vi "Helper - Best Tack Pt.vi"(10 "Point on Line":dbl[][](array[numeric]), 11 "Vector In":T1) -> (3 "Array":dbl[](array[numeric]))   [LabVIEW 2011]
uses:
  2 Typedefs/Velocity.ctl
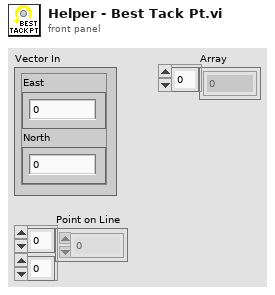
[diagram p1: front panel]
types:
  T1 = typedef "Velocity.ctl" = cluster{"East":dbl, "North":dbl}
  T2 = typedef "heading.ctl" = dbl
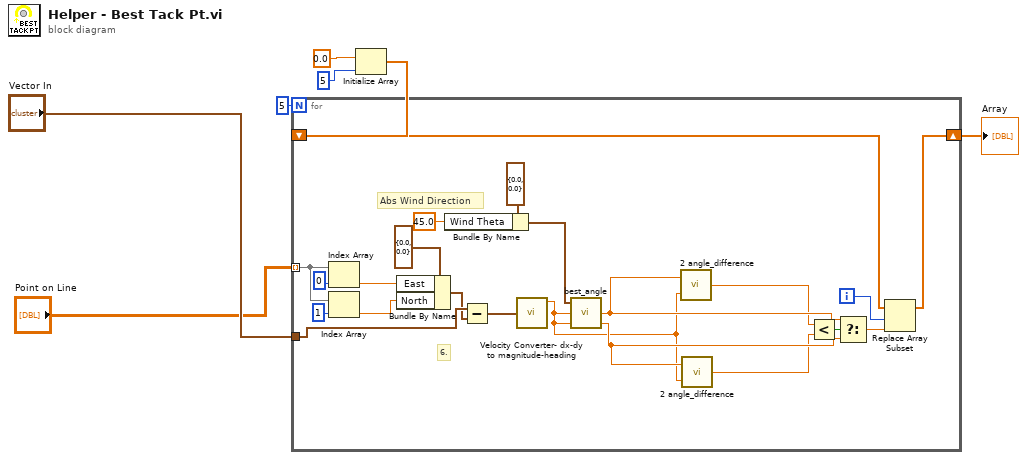
[diagram p0: block diagram]
diagram:
  n1 = Initialize Array(0.0, 5) -> (w4:dbl[])
  n2 = for {
    N: 5 -> [_]
    tunnel: "Vector In" -> [w23]
    tunnel: "Point on Line" -> [w29] mode=indexing
    shift-right: [w14] -> w5
    shift-left: w4 -> [w16]
    i -> [w15]
    # "6."
    # "Abs Wind Direction"
    n3 = Index Array(array=w29, index=0) -> (element=w25:dbl)
    n4 = Index Array(array=w29, index=1) -> (element=w24:dbl)
    n5 = Bundle By Name(cluster=T1 {"East"=0.0, "North"=0.0} ("Vector In"), "East"=w25, "North"=w24) -> (w13:T1)
    n6 = Bundle By Name(cluster=cluster{"Wind R":dbl, "Wind Theta":dbl} {"Wind R"=0.0, "Wind Theta"=0.0} ("Wind Vector"), "Wind Theta"=45.0) -> (w19:cluster{"Wind R":dbl, "Wind Theta":dbl})
    n7 = Subtract(x=w23, y=w13) -> (x-y=w22:T1)
    n8 = call "Velocity Converter- dx-dy to magnitude-heading.vi"("Vector In"=w22) -> ("Heading Out"=w9:T2)  [unwired: 9 in, 1 out]
    n9 = call "best_angle.vi"("Waypoint Heading"=w9, "Current Heading"=w9, "Wind Vector"=w19) -> ("Heading Candidate 2"=w10:dbl, "Heading Candidate 1"=w12:dbl)  [unwired: 1 out]
    n10 = call "2 angle_difference.vi"("Angle 2"=w9, "Angle 1"=w12) -> ("Difference"=w11:dbl)
    n11 = call "2 angle_difference.vi"("Angle 2"=w9, "Angle 1"=w10) -> ("Difference"=w8:dbl)
    n12 = Less?(x=w11, y=w8) -> (x < y?=w18:bool)
    n13 = Select(t=w12, s=w18, f=w10) -> (s? t:f=w17:dbl)
    n14 = Replace Array Subset(array=w16, new element=w17, index=w15) -> (w14:dbl[])
  }
  "Array" <- w5
